vi "FTW-Endpoint-ConnectToListener.vi"(0 "FTW-Endpoint In":refnum<class "FTW-Endpoint.lvclass">, 5 "Address":string, 9 "Timeout":i32=1000 format="%dmsec", 11 "error in":errorcluster) -> (4 "FTW-Endpoint Out":refnum<class "FTW-Endpoint.lvclass">, 6 "Actual Address":string, 15 "error out":errorcluster)   [LabVIEW 2013, in "FTW-Endpoint.lvclass"]
uses:
  FTW-Endpoint.lvclass
  Payload/FTW-MessagePayload.ctl
  FTW-Endpoint.lvclass/FTW-Endpoint.ctl
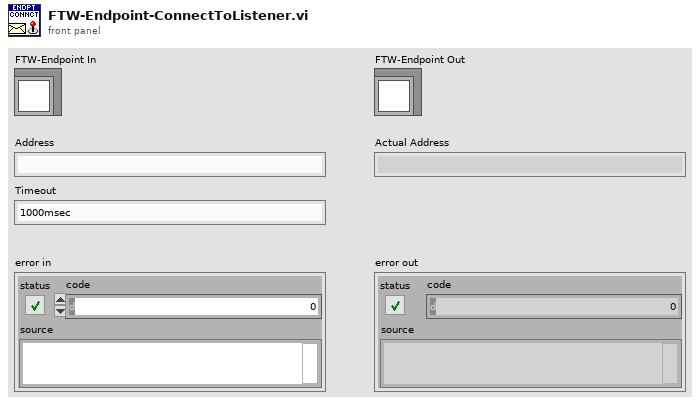
[diagram p1: front panel]
types:
  T1 = typedef "FTW-MessagePayload.ctl" = cluster{"Header":string, "Body":string, "FTW: Sender Identity":string, "FTW: Reply Address":string, "FTW: Reply Error":errorcluster}
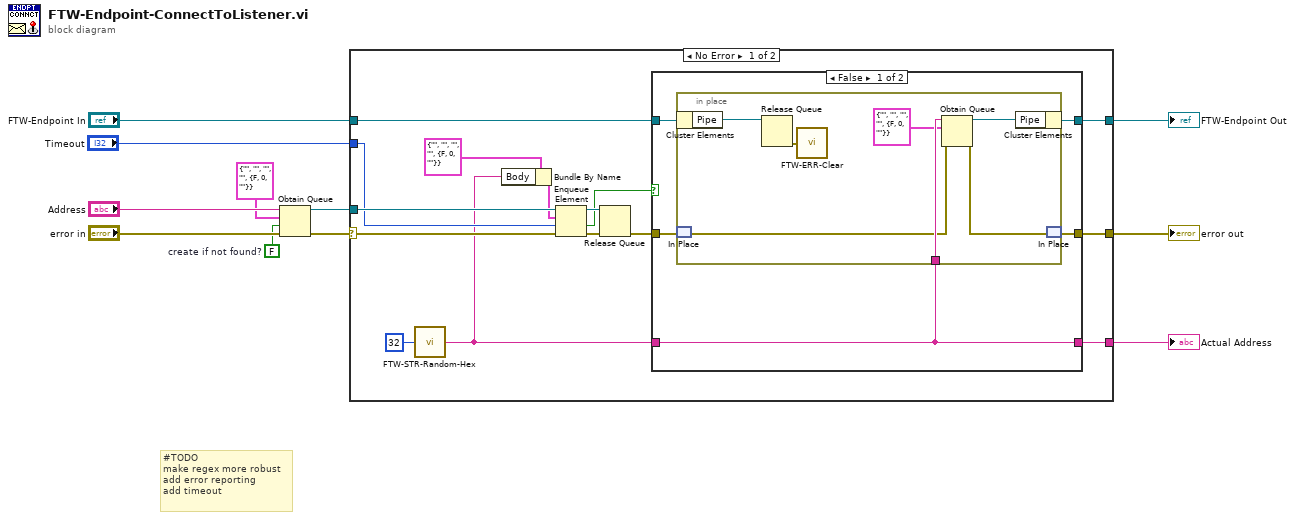
[diagram p0: block diagram]
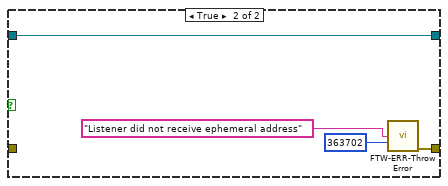
[diagram p2: hidden frame]
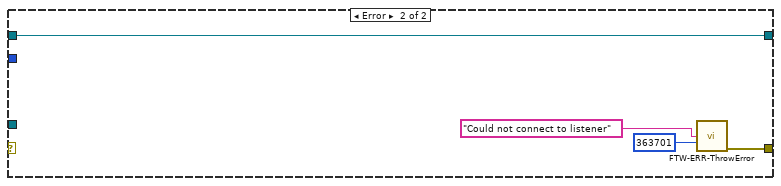
[diagram p3: hidden frame]
diagram:
  w2 = FALSE  # create if not found?
  # "#TODO\nmake regex more robust\nadd error reporting\nadd timeout"
  n1 = Obtain Queue(name (unnamed)="Address", element data type=T1 {"Header"="", "Body"="", "FTW: Sender Identity"="", "FTW: Reply Address"="", "FTW: Reply Error"={"status"=FALSE, "code"=0, "source"=""}}, create if not found? (T)=w2, error in (no error)="error in") -> (queue out=w3:refnum<queue>, error out=w4:errorcluster)  [unwired: 1 in, 1 out]
  n2 = case shown="No Error" w4 {
    selector: w4 -> [w21 _]
    tunnel: "FTW-Endpoint In" -> [w25 w46]
    tunnel: [w24 w43] -> w11
    tunnel: [w23 w46] -> w10
    tunnel: [w22 _] -> w6
    tunnel: w3 -> [w19 _]
    tunnel: "Timeout" -> [w16 _]
    frame No Error {
      n3 = call "FTW-STR-Random-Hex.vi"("String Length"=32) -> ("Random Hex String"=w13:string)  [unwired: 3 in]
      n4 = Bundle By Name(cluster=T1 {"Header"="", "Body"="", "FTW: Sender Identity"="", "FTW: Reply Address"="", "FTW: Reply Error"={"status"=FALSE, "code"=0, "source"=""}}, "Body"=w13) -> (w12:T1)
      n5 = Enqueue Element(queue=w19, element=w12, timeout in ms (-1)=w16, error in (no error)=w21) -> (queue out=w18:refnum<queue>, timed out?=w15:bool, error out=w20:errorcluster)
      n6 = Release Queue(queue=w18, error in (no error)=w20) -> (error out=w26:errorcluster)  [unwired: 1 in, 2 out]
      n7 = case shown="False" w15 {
        tunnel: w26 -> [w28 _]
        tunnel: w25 -> [w31 w42]
        tunnel: [w27 w41] -> w24
        tunnel: [w30 w42] -> w23
        tunnel: w13 -> [w29 _]
        tunnel: [w29 _] -> w22
        frame False {
          n8 = in-place {
            in-place-border: w29 -> [w35]
            n9 = in-place-cluster #1(w31) -> ("Pipe"=w38:refnum<queue>)
            n10 = in-place-match #2(w28) -> (w34:errorcluster)
            n11 = Release Queue(queue=w38) -> (error out=w37:errorcluster)  [unwired: 2 in, 2 out]
            n12 = call "FTW-ERR-Clear.vi"("error to snuff"=w37) -> ()  [unwired: 1 out]
            n13 = Obtain Queue(name (unnamed)=w35, element data type=T1 {"Header"="", "Body"="", "FTW: Sender Identity"="", "FTW: Reply Address"="", "FTW: Reply Error"={"status"=FALSE, "code"=0, "source"=""}} ("Message"), error in (no error)=w34) -> (queue out=w36:refnum<queue>, error out=w33:errorcluster)  [unwired: 2 in, 1 out]
            n14 = in-place-cluster #1("Pipe"=w36) -> (w30:refnum<class "FTW-Endpoint.lvclass">)
            n15 = in-place-match #2(w33) -> (w27:errorcluster)
          }
        }
        frame True {
          n16 = call "FTW-ERR-ThrowError.vi"("Error Message"="Listener did not receive ephemeral address", "Error Code"=363702) -> ("error out"=w41:errorcluster)  [unwired: 13 in]
        }
      }
    }
    frame Error {
      n17 = call "FTW-ERR-ThrowError.vi"("Error Message"="Could not connect to listener", "Error Code"=363701) -> ("error out"=w43:errorcluster)  [unwired: 13 in]
    }
  }
  "FTW-Endpoint Out" <- w10
  "error out" <- w11
  "Actual Address" <- w6
